vi "Read Machine Interface Opcodes_MI.vi"(7 "error in (no error)":errorcluster, 10 "Machine Interface Parameters File Path":path=path "C:/Users/veenaj/Desktop/ZenGage V1.3/Configuration file/Machine Interface Parameters.json") -> (0 "error out":errorcluster, 3 "MachineInterfaceParameters":T1)   [LabVIEW 2019, in "Machine Interface.lvclass"]
uses:
  Machine Interface.lvclass
  Controls/Machine Interface Config File Structure_MI.ctl
panel:
  in  "MachineInterfaceParameters":T1
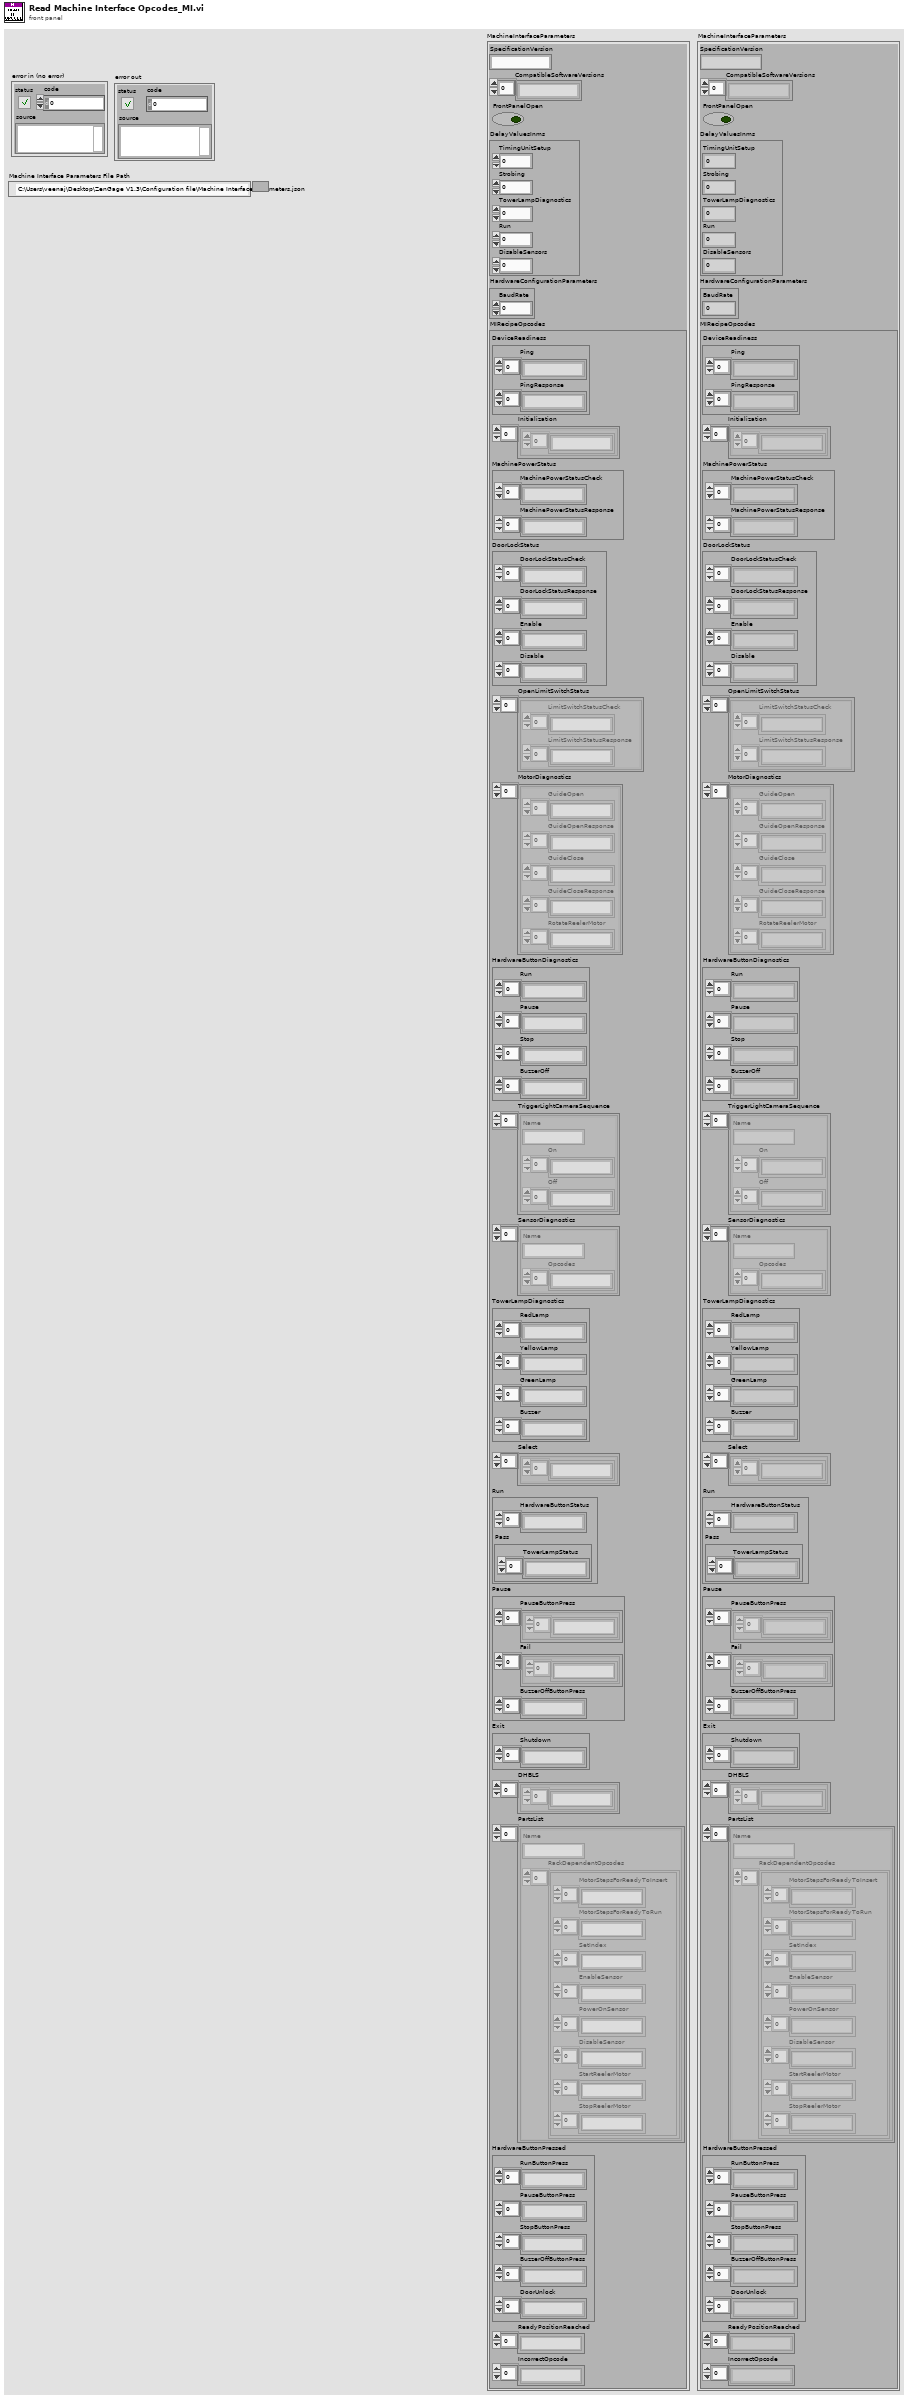
[diagram p1: front panel]
types:
  T1 = typedef "Machine Interface.lvclass/Machine Interface Config File Structure_MI.ctl" = cluster{"SpecificationVersion":string, "CompatibleSoftwareVersions":string[], "FrontPanelOpen":bool, "DelayValuesInms":cluster{"TimingUnitSetup":i32, "Strobing":i32, "TowerLampDiagnostics":i32, "Run":i32, "DisableSensors":i32}, "HardwareConfigurationParameters":cluster{"BaudRate":dbl}, "MIRecipeOpcodes":cluster{"DeviceReadiness":cluster{"Ping":string[], "PingResponse":string[]}, "Initialization":cluster{string[]}[], "MachinePowerStatus":cluster{"MachinePowerStatusCheck":string[], "MachinePowerStatusResponse":string[]}, "DoorLockStatus":cluster{"DoorLockStatusCheck":string[], "DoorLockStatusResponse":string[], "Enable":string[], "Disable":string[]}, "OpenLimitSwitchStatus":cluster{"LimitSwitchStatusCheck":string[], "LimitSwitchStatusResponse":string[]}[], "MotorDiagnostics":cluster{"GuideOpen":string[], "GuideOpenResponse":string[], "GuideClose":string[], "GuideCloseResponse":string[], "RotateReelerMotor":string[]}[], "HardwareButtonDiagnostics":cluster{"Run":string[], "Pause":string[], "Stop":string[], "BuzzerOff":string[]}, "TriggerLightCameraSequence":cluster{"Name":string, "On":string[], "Off":string[]}[], "SensorDiagnostics":cluster{"Name":string, "Opcodes":string[]}[], "TowerLampDiagnostics":cluster{"RedLamp":string[], "YellowLamp":string[], "GreenLamp":string[], "Buzzer":string[]}, "Select":cluster{string[]}[], "Run":cluster{"HardwareButtonStatus":string[], "Pass":cluster{"TowerLampStatus":string[]}}, "Pause":cluster{"PauseButtonPress":cluster{string[]}[], "Fail":cluster{string[]}[], "BuzzerOffButtonPress":string[]}, "Exit":cluster{"Shutdown":string[]}, "DHBLS":cluster{string[]}[], "PartsList":cluster{"Name":string, "RackDependentOpcodes":cluster{"MotorStepsForReadyToInsert":string[], "MotorStepsForReadyToRun":string[], "SetIndex":string[], "EnableSensor":string[], "PowerOnSensor":string[], "DisableSensor":string[], "StartReelerMotor":string[], "StopReelerMotor":string[]}[]}[], "HardwareButtonPressed":cluster{"RunButtonPress":string[], "PauseButtonPress":string[], "StopButtonPress":string[], "BuzzerOffButtonPress":string[], "DoorUnlock":string[]}, "ReadyPositionReached":string[], "IncorrectOpcode":string[]}}
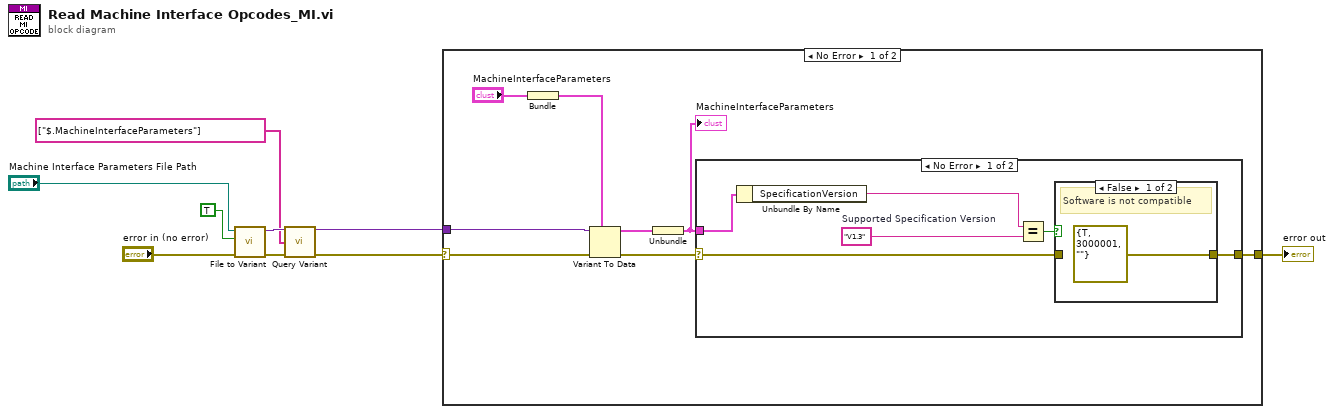
[diagram p0: block diagram]
diagram:
  n1 = call <vilib>:"File to Variant.vi"("JSON FilePath"="Machine Interface Parameters File Path", "Remove Comments?"=TRUE, "error in (no error)"="error in (no error)") -> ("JSON Variant"=w6:variant, "error out"=w3:errorcluster)  [unwired: 5 in, 1 out]
  n2 = call <vilib>:"Query Variant.vi"("VCluster in"=w6, "pathList"=string[] ["$.MachineInterfaceParameters"], "error IO"=w3) -> ("VCluster\n out"=w4:variant, "error out"=w1:errorcluster)  [unwired: 9 in, 2 out]
  n3 = case shown="No Error" w1 {
    selector: w1 -> [w13 w27]
    tunnel: w4 -> [w17 _]
    tunnel: [w14 w27] -> w2
    frame No Error {
      n4 = Bundle("MachineInterfaceParameters"="MachineInterfaceParameters") -> (w11:cluster{"MachineInterfaceParameters":T1})  [unwired: 1 in]
      n5 = Variant To Data(error in=w13, type=w11, Variant=w17) -> (data=w16:cluster{"MachineInterfaceParameters":T1}, error out=w15:errorcluster)
      n6 = Unbundle(w16) -> ("MachineInterfaceParameters"=w10:T1)
      "MachineInterfaceParameters" <- w10
      n7 = case shown="No Error" w15 {
        selector: w15 -> [w18 w26]
        tunnel: w10 -> [w23 _]
        tunnel: [w19 w26] -> w14
        frame No Error {
          w21 = "V1.3"  # Supported Specification Version
          n8 = Unbundle By Name(w23) -> ("SpecificationVersion"=w22:string)
          n9 = Equal?(x=w22, y=w21) -> (x = y?=w20:bool)
          n10 = case shown="False" w20 {
            tunnel: [errorcluster {"status"=TRUE, "code"=3000001, "source"=""} ("error IO") w25] -> w19
            tunnel: w18 -> [_ w25]
            frame False {
              # "Software is not compatible"
            }
            frame True {
              # "Software is compatible"
            }
          }
        }
        frame Error {
        }
      }
    }
    frame Error {
    }
  }
  "error out" <- w2
